vi "Data File Processing UI Find Control By Name.vi"(8 "error in (no error)":errorcluster, 9 "control name":string, 11 "vi refnum in":refnum<vi>) -> (0 "error out":errorcluster, 2 "control refnum":refnum<vi>, 3 "vi refnum out":refnum<vi>)   [LabVIEW 2011]
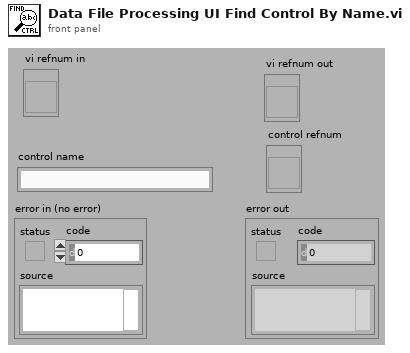
[diagram p1: front panel]
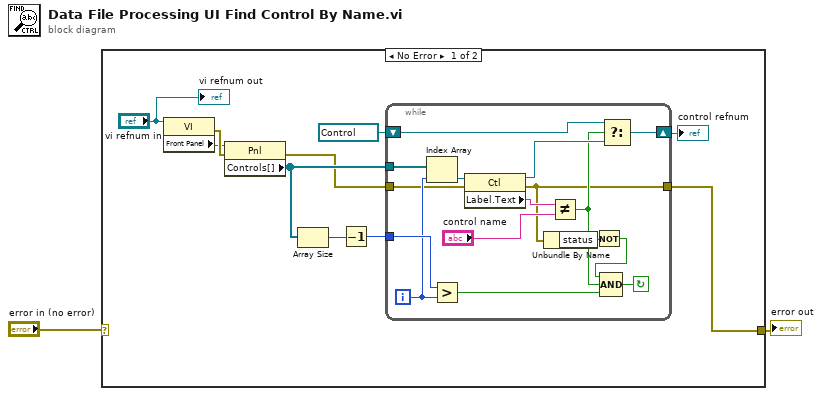
[diagram p0: block diagram]
diagram:
  n1 = case shown="No Error" "error in (no error)" {
    selector: "error in (no error)" -> [_ w29]
    tunnel: [w4 w29] -> w1
    frame No Error {
      n2 = property class="VI"(reference="vi refnum in") -> (error out=w12:errorcluster, "Front Panel"=w11:refnum<vi>)  [unwired: 1 in, 1 out]
      n3 = property class="Pnl"(reference=w11, error in=w12) -> (error out=w5:errorcluster, "Controls[]"=w9:refnum<vi>[])  [unwired: 1 out]
      n4 = Array Size(array=w9) -> (size(s)=w10:i32)
      n5 = Decrement(x=w10) -> (x-1=w6:i32)
      n6 = while {
        tunnel: w6 -> [w28]
        tunnel: w9 -> [w27]
        shift-right: [w22] -> w7
        shift-left: refnum<vi> refnum ("dup reference") -> [w21]
        tunnel: w5 -> [w16]
        tunnel: [w13] -> w4
        i -> [w26]
        stop <- w19 continue-if-true
        n7 = Index Array(array=w27, index=w26) -> (element=w25:refnum<vi>)
        n8 = Greater?(x=w28, y=w26) -> (0:w17:bool)
        n9 = property class="Ctl"(reference=w25, error in=w16) -> (reference out=w20:refnum<vi>, error out=w13:errorcluster, "Label.Text"=w24:string)
        n10 = Unbundle By Name(w13) -> ("status"=w15:bool)
        n11 = Not Equal?(x=w24, y="control name") -> (x != y?=w18:bool)
        n12 = Not(x=w15) -> (.not. x?=w14:bool)
        n13 = Compound Arithmetic op=AND(w14, w18, w17) -> (w19:bool)
        n14 = Select(t=w21, s=w18, f=w20) -> (s? t:f=w22:refnum<vi>)
      }
      "control refnum" <- w7
      "vi refnum out" <- "vi refnum in"
    }
    frame Error {
    }
  }
  "error out" <- w1
